vi "mxwScript_Cmnd2Str_setUseLibrariesToSave.vi"(8 "error in (no error)":errorcluster, 11 "data":variant) -> (0 "error out":errorcluster, 3 "outputString":string)   [LabVIEW 2020]
uses:
  codeGenAPISupport.llb/cgAPI_mxwScript_Save_OptionUseLibrariesToSaveData.ctl
  codeGenAPISupport.llb/cgAPI_mxwScript_Save_SaveInLibraryOptions.ctl
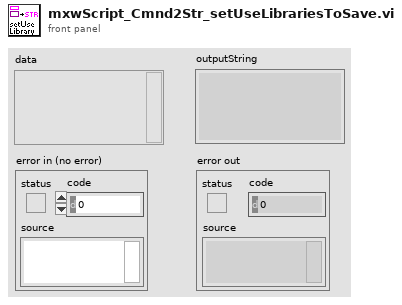
[diagram p1: front panel]
types:
  T1 = typedef "cgAPI_mxwScript_Save_OptionUseLibrariesToSaveData.ctl" = cluster{"SaveInLibrary":T2, "IconPath":path, "Name":string, "LocalizedName":string, "Description":string, "HelpPath":path, "HelpTag":string}
  T2 = typedef "cgAPI_mxwScript_Save_SaveInLibraryOptions.ctl" = enum16{"Always", "Never", "IfSubVIs"}
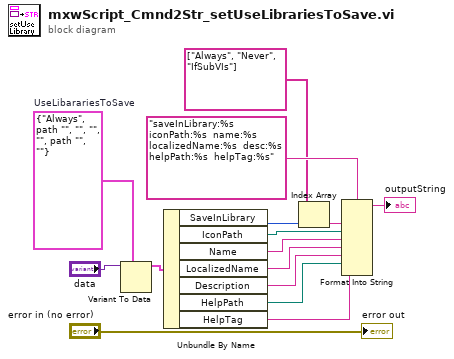
[diagram p0: block diagram]
diagram:
  w11 = T1 {"SaveInLibrary"=enum."Always", "IconPath"=path "", "Name"="", "LocalizedName"="", "Description"="", "HelpPath"=path "", "HelpTag"=""}  # UseLibarariesToSave
  n1 = Variant To Data(type=w11, Variant="data") -> (data=w13:T1)  [unwired: 1 in, 1 out]
  n2 = Unbundle By Name(w13) -> ("SaveInLibrary"=w9:T2, "IconPath"=w6:path, "Name"=w5:string, "LocalizedName"=w4:string, "Description"=w3:string, "HelpPath"=w2:path, "HelpTag"=w1:string)
  n3 = Index Array(array=string[] ["Always", "Never", "IfSubVIs"], index=w9) -> (element=w7:string)
  n4 = Format Into String(format string="saveInLibrary:%s  iconPath:%s  name:%s  localizedName:%s  desc:%s  helpPath:%s  helpTag:%s", w7, w6, w5, w4, w3, w2, w1) -> (resulting string=→"outputString":string)  [unwired: 2 in, 1 out]
  "error out" <- "error in (no error)"
